vi "Initialize Default.vi"(8 "error in":errorcluster, 11 "RDMA Rx Transfer Configuration in":refnum<class "RDMA Transfer Rx Configuration.lvclass">) -> (0 "error out":errorcluster, 3 "RDMA Rx Transfer Configuration out":refnum<class "RDMA Transfer Rx Configuration.lvclass">)   [LabVIEW 2020, in "RDMA.lvlib" / "RDMA Transfer Rx Configuration.lvclass"]
uses:
  RDMA Transfer Rx Configuration.lvclass
  Rx Transfer Settings.ctl
  RDMA Transfer Rx Configuration.lvclass/RDMA Transfer Rx Configuration.ctl
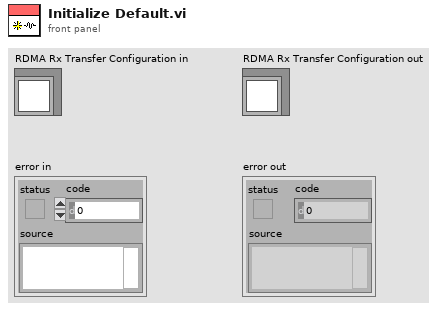
[diagram p1: front panel]
types:
  T1 = typedef "RDMA.lvlib/RDMA Transfer Rx Configuration.lvclass/Rx Transfer Settings.ctl" = cluster{"local address":u32, "local port":u16, "decimation":u16}
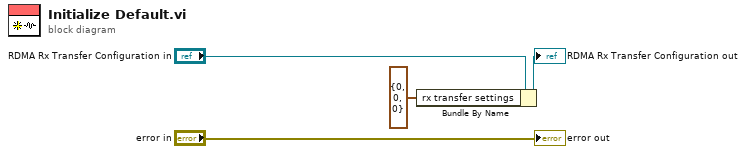
[diagram p0: block diagram]
diagram:
  n1 = Bundle By Name(cluster="RDMA Rx Transfer Configuration in", "rx transfer settings"=T1 {"local address"=0, "local port"=0, "decimation"=0}) -> (→"RDMA Rx Transfer Configuration out":refnum<class "RDMA Transfer Rx Configuration.lvclass">)
  "error out" <- "error in"
